vi "Qudi_multicolour_scan_Kinetix.vi"(3 "N Z positions":i32) -> ()   [LabVIEW 2015]
uses:
  <vilib>/rvi/Emulation/niFpgaGetClockAttributes.vi
  <vilib>/rvi/Emulation/niFpgaSctlEmulationGetInTimedLoop.vi
  <vilib>/rvi/Emulation/niFpgaEmulationReportErrorSimple.vi
  <vilib>/rvi/eio/common/nirviEmuTemplateMethod_errors.vi
  <vilib>/rvi/Emulation/niFpgaProcessEmulError.vi
  <vilib>/rvi/Emulation/niFpgaCriticalErrorInLSC.vi
  <vilib>/eio/EIONode/EIONode.xnode
panel:
  in  "exposure_time_ms":u16
  in  "stop":bool
  out "n cycles":i32
  out "Images acquired":i32
  in  "Laser lines":i32[](array[numeric])=[0, 0, 0, 0, 0, 0, 0, 0, 0, 0]
  in  "N laser lines":i32
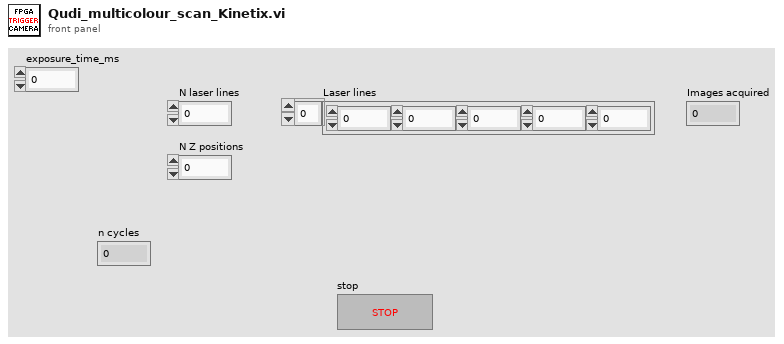
[diagram p1: front panel]
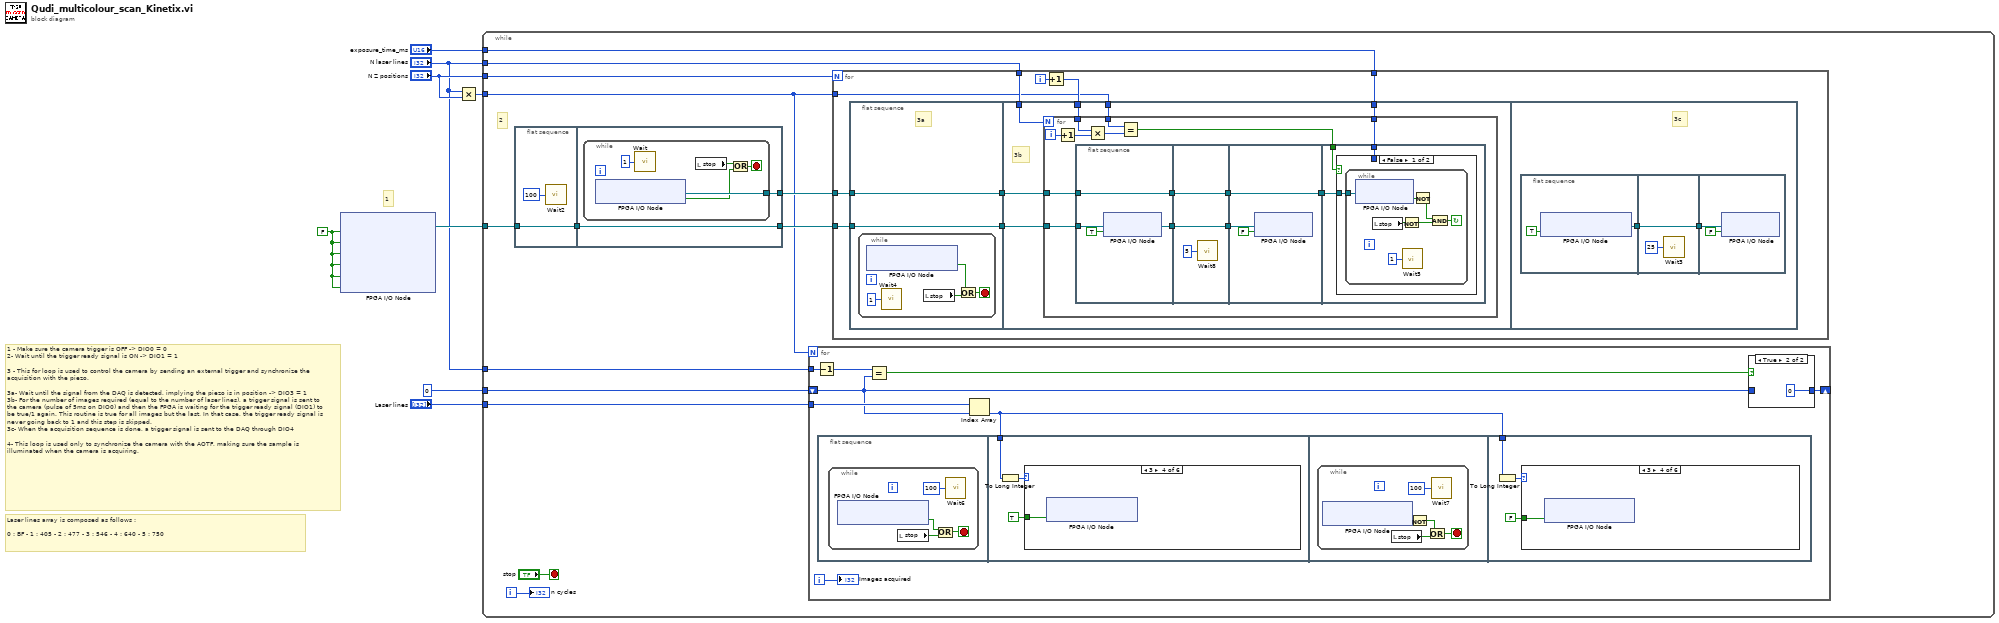
[diagram p0: block diagram]
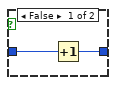
[diagram p2: hidden frame]
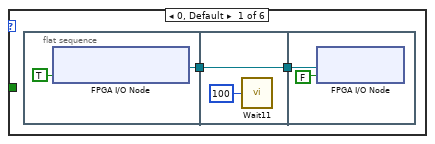
[diagram p3: hidden frame]
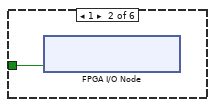
[diagram p4: hidden frame]
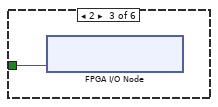
[diagram p5: hidden frame]
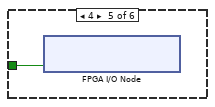
[diagram p6: hidden frame]
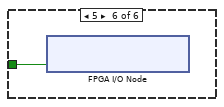
[diagram p7: hidden frame]
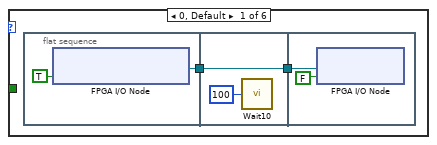
[diagram p8: hidden frame]
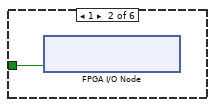
[diagram p9: hidden frame]
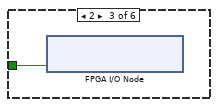
[diagram p10: hidden frame]
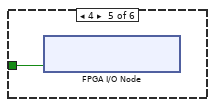
[diagram p11: hidden frame]
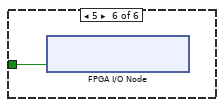
[diagram p12: hidden frame]
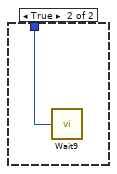
[diagram p13: hidden frame]
diagram:
  w1 = FALSE ("Connector0/DIO0")
  # "Laser lines array is composed as follows :\n\n0 : BF - 1 : 405 - 2 : 477 - 3 : 546 - 4 : 640 - 5 : 750"
  # "1"
  # "1 - Make sure the camera trigger is OFF -> DIO0 = 0\n2- Wait until the trigger ready signal is ON -> DIO1 = 1\n\n3 - This for loop is used to control the camera by sending an external trigger and synchronize the acquisition with the piezo.\n\n3a- Wait until the signal from the DAQ is detected, implying the piezo is in position -> DIO3 = 1 \n3b- For the number of images required (equal to the number of laser lines), a trigger signal is sent to the camera (pulse of 5ms on DIO0) and then the FPGA is waiting for the trigger ready signal (DIO1) to be true/1 again. This routine is true for all images but the last. In that case, the trigger ready signal is never going back to 1 and this step is skipped. \n3c- When the acquisition sequence is done, a trigger signal is sent to the DAQ through DIO4\n\n4- This loop is used only to synchronize the camera with the AOTF, making sure the sample is illuminated when the camera is acquiring."
  n1 = xnode "FPGA I/O Node"("Connector0/DIO0"=w1, "Connector0/DIO6"=w1, "Connector0/DIO7"=w1, "Connector0/DIO8"=w1, "Connector0/DIO9"=w1, "Connector0/DIO10"=w1) -> ("FPGA I/O Out"=w8:refnum<k21>)  [unwired: 6 in, 5 out]
  n2 = Multiply(x="N laser lines", y="N Z positions") -> (x*y=w4:i32)
  n3 = while {
    tunnel: w8 -> [w20]
    tunnel: "Laser lines" -> [w17]
    tunnel: 0 -> [w16]
    tunnel: "N Z positions" -> [w15]
    tunnel: "N laser lines" -> [w13]
    tunnel: w4 -> [w12]
    tunnel: "N laser lines" -> [w11]
    tunnel: "exposure_time_ms" -> [w10]
    i -> [w14]
    stop <- "stop" stop-if-true
    # "2"
    n4 = flat-sequence {
      tunnel: w20 -> [w75]
      tunnel: [w75] -> w21
      tunnel: w21 -> [w77]
      tunnel: [w77] -> w19
      tunnel: [w76] -> w18
      frame #0 {
        n5 = call "Wait2"("Count(uSec)"=u8 100 ("Count(mSec)")) -> ()  [unwired: 1 out]
      }
      frame #1 {
        n6 = while {
          tunnel: [w82] -> w76
          stop <- w80 stop-if-true
          n7 = xnode "FPGA I/O Node"() -> ("Connector0/DIO1"=w78:bool, "FPGA I/O Out"=w82:refnum<k21>)  [unwired: 1 in]
          n8 = call "Wait"("Count(mSec)"=u8 1) -> ()  [unwired: 1 out]
          n9 = local read "stop"() -> (w81:bool)
          n10 = Or(x=w81, y=w78) -> (x .or. y?=w80:bool)
        }
      }
    }
    n11 = for {
      N: w12 -> [_]
      shift-right: [w27] -> _
      shift-left: w16 -> [w25]
      tunnel: w17 -> [w26]
      tunnel: w11 -> [w24]
      i -> [w22]
      n12 = Decrement(x=w24) -> (x-1=w23:i32)
      n13 = flat-sequence {
        tunnel: w29 -> [w38]
        tunnel: w29 -> [w58]
        frame #0 {
          n14 = while {
            stop <- w35 stop-if-true
            n15 = xnode "FPGA I/O Node"() -> ("Connector0/DIO2"=w36:bool)  [unwired: 1 in, 1 out]
            n16 = local read "stop"() -> (w33:bool)
            n17 = Or(x=w36, y=w33) -> (x .or. y?=w35:bool)
            n18 = call "Wait6"("Count(uSec)"=u8 100 ("Count(mSec)")) -> ()  [unwired: 1 out]
          }
        }
        frame #1 {
          n19 = To Long Integer(number=w38) -> (32bit integer=w39:i32)
          n20 = case shown="3" w39 {
            tunnel: TRUE ("Connector0/DIO6") -> [_ w48 w49 w50 w51 w52]
            frame 0, Default {
              n21 = flat-sequence {
                tunnel: [w42] -> w41
                tunnel: w41 -> [w44]
                tunnel: [w44] -> w40
                tunnel: w40 -> [w47]
                frame #0 {
                  n22 = xnode "FPGA I/O Node"("Connector0/DIO5"=TRUE) -> ("FPGA I/O Out"=w42:refnum<k21>)  [unwired: 1 in]
                }
                frame #1 {
                  n23 = call "Wait11"("Count(uSec)"=u32 100) -> ()  [unwired: 1 out]
                }
                frame #2 {
                  n24 = xnode "FPGA I/O Node"("I/O Item"=FALSE, "FPGA I/O In"=w47) -> ()  [unwired: 1 out]
                }
              }
            }
            frame 1 {
              n25 = xnode "FPGA I/O Node"("Connector0/DIO8"=w48) -> ()  [unwired: 1 in, 1 out]
            }
            frame 2 {
              n26 = xnode "FPGA I/O Node"("Connector0/DIO9"=w49) -> ()  [unwired: 1 in, 1 out]
            }
            frame 3 {
              n27 = xnode "FPGA I/O Node"("Connector0/DIO6"=w50) -> ()  [unwired: 1 in, 1 out]
            }
            frame 4 {
              n28 = xnode "FPGA I/O Node"("Connector0/DIO7"=w51) -> ()  [unwired: 1 in, 1 out]
            }
            frame 5 {
              n29 = xnode "FPGA I/O Node"("Connector0/DIO10"=w52) -> ()  [unwired: 1 in, 1 out]
            }
          }
        }
        frame #2 {
          n30 = while {
            stop <- w55 stop-if-true
            n31 = xnode "FPGA I/O Node"() -> ("Connector0/DIO2"=w56:bool)  [unwired: 1 in, 1 out]
            n32 = local read "stop"() -> (w57:bool)
            n33 = Not(x=w56) -> (.not. x?=w53:bool)
            n34 = Or(x=w53, y=w57) -> (x .or. y?=w55:bool)
            n35 = call "Wait7"("Count(uSec)"=u8 100 ("Count(mSec)")) -> ()  [unwired: 1 out]
          }
        }
        frame #3 {
          n36 = To Long Integer(number=w58) -> (32bit integer=w59:i32)
          n37 = case shown="3" w59 {
            tunnel: FALSE ("Connector0/DIO6") -> [_ w69 w70 w71 w72 w73]
            frame 0, Default {
              n38 = flat-sequence {
                tunnel: [w63] -> w62
                tunnel: w62 -> [w65]
                tunnel: [w65] -> w61
                tunnel: w61 -> [w68]
                frame #0 {
                  n39 = xnode "FPGA I/O Node"("Connector0/DIO5"=TRUE) -> ("FPGA I/O Out"=w63:refnum<k21>)  [unwired: 1 in]
                }
                frame #1 {
                  n40 = call "Wait10"("Count(uSec)"=u32 100) -> ()  [unwired: 1 out]
                }
                frame #2 {
                  n41 = xnode "FPGA I/O Node"("I/O Item"=FALSE, "FPGA I/O In"=w68) -> ()  [unwired: 1 out]
                }
              }
            }
            frame 1 {
              n42 = xnode "FPGA I/O Node"("Connector0/DIO8"=w69) -> ()  [unwired: 1 in, 1 out]
            }
            frame 2 {
              n43 = xnode "FPGA I/O Node"("Connector0/DIO9"=w70) -> ()  [unwired: 1 in, 1 out]
            }
            frame 3 {
              n44 = xnode "FPGA I/O Node"("Connector0/DIO6"=w71) -> ()  [unwired: 1 in, 1 out]
            }
            frame 4 {
              n45 = xnode "FPGA I/O Node"("Connector0/DIO7"=w72) -> ()  [unwired: 1 in, 1 out]
            }
            frame 5 {
              n46 = xnode "FPGA I/O Node"("Connector0/DIO10"=w73) -> ()  [unwired: 1 in, 1 out]
            }
          }
        }
      }
      n47 = Equal?(x=w23, y=w25) -> (x = y?=w28:bool)
      n48 = Index Array(array=w26, index=w25) -> (element=w29:i32)
      n49 = case shown="True" w28 {
        tunnel: w25 -> [w31 _]
        tunnel: [w30 0] -> w27
        frame False {
          n50 = Increment(x=w31) -> (x+1=w30:i32)
        }
        frame True {
        }
      }
      "Images acquired" <- w22
    }
    n51 = for {
      N: w15 -> [_]
      tunnel: w19 -> [w90]
      tunnel: w18 -> [w91]
      tunnel: w13 -> [w86]
      tunnel: w12 -> [w84]
      tunnel: w10 -> [w83]
      i -> [w87]
      n52 = flat-sequence {
        tunnel: w90 -> [w92]
        tunnel: w91 -> [w93]
        tunnel: [w93] -> w89
        tunnel: [w92] -> w88
        tunnel: w89 -> [w103]
        tunnel: w88 -> [w102]
        tunnel: w86 -> [w101]
        tunnel: w85 -> [w100]
        tunnel: w84 -> [w99]
        tunnel: w83 -> [w98]
        frame #0 {
          # "3a"
          n53 = while {
            stop <- w95 stop-if-true
            n54 = xnode "FPGA I/O Node"() -> ("Connector0/DIO3"=w96:bool)  [unwired: 1 in, 1 out]
            n55 = call "Wait4"("Count(mSec)"=u8 1) -> ()  [unwired: 1 out]
            n56 = local read "stop"() -> (w97:bool)
            n57 = Or(x=w96, y=w97) -> (x .or. y?=w95:bool)
          }
        }
        frame #1 {
          # "3b"
          n58 = for {
            N: w101 -> [_]
            tunnel: w103 -> [w112]
            tunnel: w102 -> [w111]
            tunnel: w100 -> [w108]
            tunnel: w99 -> [w106]
            tunnel: w98 -> [w104]
            i -> [w110]
            n59 = Increment(x=w110) -> (x+1=w109:i32)
            n60 = flat-sequence {
              tunnel: [w120] -> w117
              tunnel: [w118] -> w116
              tunnel: w111 -> [w119]
              tunnel: w112 -> [w118]
              tunnel: w117 -> [w124]
              tunnel: [w124] -> w115
              tunnel: [w123] -> w114
              tunnel: w116 -> [w123]
              tunnel: w115 -> [w126]
              tunnel: [w125] -> w113
              tunnel: w114 -> [w125]
              tunnel: w113 -> [w130]
              tunnel: w105 -> [w129]
              tunnel: w104 -> [w128]
              frame #0 {
                n61 = xnode "FPGA I/O Node"("I/O Item"=TRUE ("Connector0/DIO0"), "FPGA I/O In"=w119) -> ("FPGA I/O Out"=w120:refnum<k21>)
              }
              frame #1 {
                n62 = call "Wait8"("Count(mSec)"=u8 5) -> ()  [unwired: 1 out]
              }
              frame #2 {
                n63 = xnode "FPGA I/O Node"("I/O Item"=FALSE ("Connector0/DIO0"), "FPGA I/O In"=w126) -> ()  [unwired: 1 out]
              }
              frame #3 {
                n64 = case shown="False" w129 {
                  tunnel: w130 -> [w131 _]
                  tunnel: w128 -> [_ w139]
                  frame False {
                    n65 = while {
                      tunnel: w131 -> [w138]
                      stop <- w134 continue-if-true
                      n66 = xnode "FPGA I/O Node"("FPGA I/O In"=w138) -> ("I/O Item"=w135:bool)  [unwired: 1 out]
                      n67 = local read "stop"() -> (w137:bool)
                      n68 = Not(x=w137) -> (.not. x?=w136:bool)
                      n69 = call "Wait5"("Count(mSec)"=u8 1) -> ()  [unwired: 1 out]
                      n70 = Not(x=w135) -> (.not. x?=w132:bool)
                      n71 = And(x=w132, y=w136) -> (x .and. y?=w134:bool)
                    }
                  }
                  frame True {
                    n72 = call "Wait9"("Count(mSec)"=w139) -> ()  [unwired: 1 out]
                  }
                }
              }
            }
            n73 = Multiply(x=w108, y=w109) -> (x*y=w107:i32)
            n74 = Equal?(x=w106, y=w107) -> (x = y?=w105:bool)
          }
        }
        frame #2 {
          # "3c"
          n75 = flat-sequence {
            tunnel: [w143] -> w141
            tunnel: w141 -> [w144]
            tunnel: [w144] -> w140
            tunnel: w140 -> [w146]
            frame #0 {
              n76 = xnode "FPGA I/O Node"("Connector0/DIO4"=TRUE) -> ("FPGA I/O Out"=w143:refnum<k21>)  [unwired: 1 in]
            }
            frame #1 {
              n77 = call "Wait3"("Count(mSec)"=u8 25) -> ()  [unwired: 1 out]
            }
            frame #2 {
              n78 = xnode "FPGA I/O Node"("I/O Item"=FALSE ("Connector0/DIO0"), "FPGA I/O In"=w146) -> ()  [unwired: 1 out]
            }
          }
        }
      }
      n79 = Increment(x=w87) -> (x+1=w85:i32)
    }
    "n cycles" <- w14
  }
